vi "get_curr_position.vi"(8 "error in (no error)":errorcluster, 11 "dummyStage in":refnum<class "dummyStage.lvclass">) -> (0 "error out":errorcluster, 2 "readback position":dbl[](array[numeric]), 3 "dummyStage out":refnum<class "dummyStage.lvclass">)   [LabVIEW 2019, in "dummyStage.lvlib" / "dummyStage.lvclass"]
uses:
  dummyStage.lvclass
  _stage/_stage.lvlibp/_stageClass/_stage.lvclass
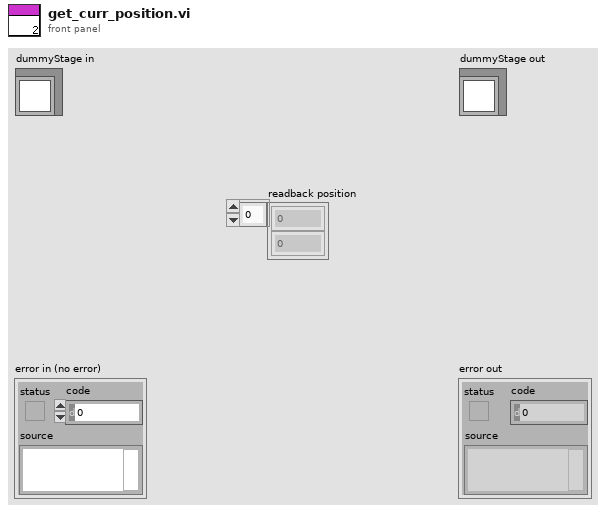
[diagram p1: front panel]
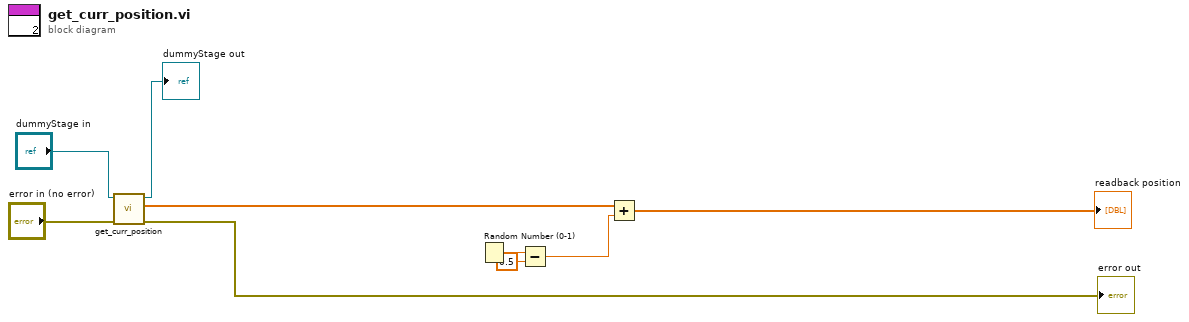
[diagram p0: block diagram]
diagram:
  n1 = call-parent "get_curr_position.vi"("error in (no error)"="error in (no error)", "_stage in"="dummyStage in") -> ("error out"=→"error out":errorcluster, "readback position"=w3:dbl[], "_stage out"=→"dummyStage out":refnum<class "dummyStage.lvclass">)  [unwired: 7 in]
  n2 = Random Number (0-1)() -> (number: 0 to 1=w5:dbl)
  n3 = Subtract(x=w5, y=0.5) -> (x-y=w2:dbl)
  n4 = Add(x=w3, y=w2) -> (x+y=→"readback position":dbl[])
